vi "Wrap Point (Zero To Max).vi"(10 "Max":T1, 11 "Point":T1) -> (3 "Point (Wrapped)":T1)   [LabVIEW 2018, in "Math.lvlib"]
uses:
  Math.lvlib
  LabSDL2/Source/Libraries/SDL2 Utility/Point (I32).ctl
  LabSDL2/Source/Libraries/SDL2 Utility/SDL2 Utility.lvlib
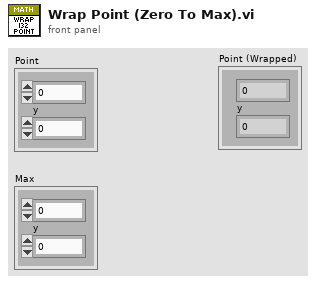
[diagram p1: front panel]
types:
  T1 = typedef "SDL2 Utility.lvlib/Point (I32).ctl" = cluster{"x":i32, "y":i32}
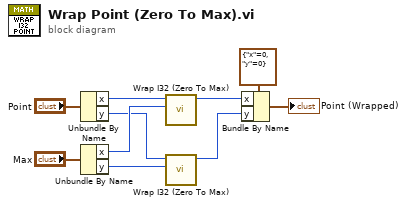
[diagram p0: block diagram]
diagram:
  n1 = Unbundle By Name("Point") -> ("x"=w8:i32, "y"=w1:i32)
  n2 = Unbundle By Name("Max") -> ("x"=w7:i32, "y"=w4:i32)
  n3 = call "Wrap I32 (Zero To Max).vi"("Max"=w7, "Value"=w8) -> ("Wrapped"=w2:i32)  [unwired: 9 in]
  n4 = call "Wrap I32 (Zero To Max).vi"("Max"=w4, "Value"=w1) -> ("Wrapped"=w3:i32)  [unwired: 9 in]
  n5 = Bundle By Name(cluster=T1 {"x"=0, "y"=0} ("World Position (Wrapped)"), "x"=w2, "y"=w3) -> (→"Point (Wrapped)":T1)
